vi "Tactic_v2_Init.vi"(0 "object in":refnum<class "Tactic_v2.lvclass">, 5 "error in (no error)":errorcluster) -> (14 "object out":refnum<class "Tactic_v2.lvclass">, 19 "error out":errorcluster)   [LabVIEW 2023, in "Tactic_v2.lvclass"]
uses:
  Tactic_v2.lvclass
  Tactic_v2.lvclass/Tactic_v2.ctl
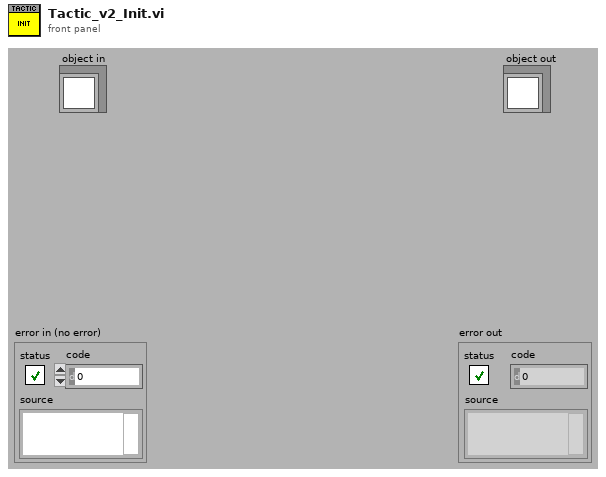
[diagram p1: front panel]
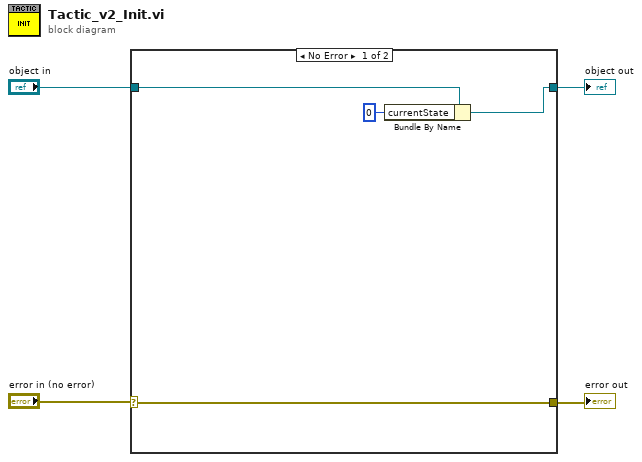
[diagram p0: block diagram]
diagram:
  n1 = case shown="No Error" "error in (no error)" {
    selector: "error in (no error)" -> [w8 w9]
    tunnel: "object in" -> [w7 w10]
    tunnel: [w6 w10] -> w3
    tunnel: [w8 w9] -> w1
    frame No Error {
      n2 = Bundle By Name(cluster=w7, "currentState"=u8 0) -> (w6:refnum<class "Tactic_v2.lvclass">)
    }
    frame Error {
    }
  }
  "object out" <- w3
  "error out" <- w1
